vi "Process Return Value.vi"(10 "Method VI":refnum<vi>, 11 "Enum Writer in":refnum<class "Enum Writer.lvclass">) -> (2 "Modified Proto Method  VI":refnum<vi>, 3 "Enum Writer out":refnum<class "Enum Writer.lvclass">)   [LabVIEW 2013, in "Enum Writer.lvclass"]
uses:
  Enum Writer.lvclass
  Enum Writer.lvclass/Enum Writer.ctl
  Abstract Param Writer/Abstract Param Writer.lvclass
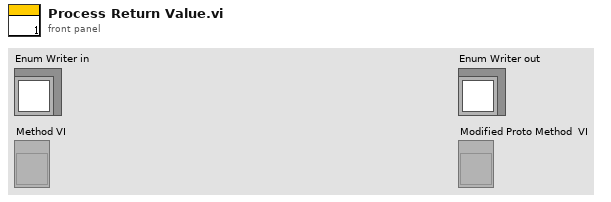
[diagram p1: front panel]
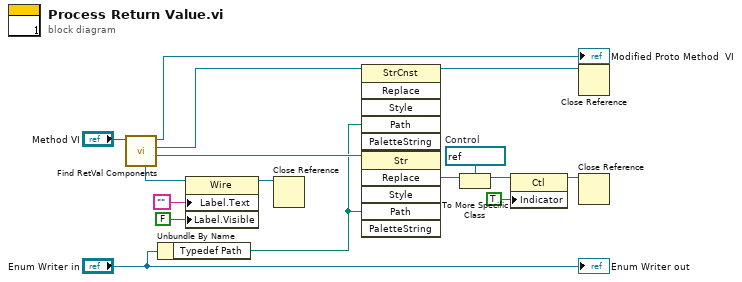
[diagram p0: block diagram]
diagram:
  w6 = refnum<vi> refnum  # Control
  n1 = call "Find RetVal Components.vi"("Proto Method VI"="Method VI") -> ("Indicator"=w12:refnum<vi>, "Data Buffer"=w14:refnum<vi>, "Proto Method VI Dup"=→"Modified Proto Method  VI":refnum<vi>, "Wire"=w1:refnum<vi>)  [unwired: 6 in, 1 out]
  n2 = Unbundle By Name("Enum Writer in") -> ("Typedef Path"=w11:path)
  n3 = property class="Wire"(reference=w1, "Label.Text"="", "Label.Visible"=FALSE) -> (reference out=w3:refnum<vi>)  [unwired: 1 in, 1 out]
  n4 = Close Reference(reference=w3) -> ()  [unwired: 1 in, 1 out]
  n5 = invoke class="StrCnst" method="Replace"(reference=w14, "Path"=w11) -> (reference out=w10:refnum<vi>)  [unwired: 4 in, 5 out]
  n6 = invoke class="Str" method="Replace"(reference=w12, "Path"=w11) -> ("Replace"=w8:refnum<vi>)  [unwired: 4 in, 5 out]
  n7 = To More Specific Class(target class=w6, reference=w8) -> (specific class reference=w7:refnum<vi>)  [unwired: 1 in, 1 out]
  n8 = property class="Ctl"(reference=w7, "Indicator"=TRUE) -> (reference out=w5:refnum<vi>)  [unwired: 1 in, 1 out]
  n9 = Close Reference(reference=w10) -> ()  [unwired: 1 in, 1 out]
  n10 = Close Reference(reference=w5) -> ()  [unwired: 1 in, 1 out]
  "Enum Writer out" <- "Enum Writer in"
